vi "XIPIN_FIFO_Generator_13_0.vi"   [LabVIEW 2017]
doc: "The FIFO Generator is a parameterizable first-in/first-out memory queue generator. Use it to generate resource and performance optimized FIFOs with common or independent read/write clock domains, and optional fixed or programmable full and empty flags and handshaking signals. Choose from a selection of memory resource types for implementation. Optional Hamming code based error detection and correction as well as error injection capability for system test help to insure data integrity. FIFO width and depth are parameterizable, and for native interface FIFOs, asymmetric read and write port widths are also supported.\n------------------------------------\n<b>Need License</b> : No\n<b>Interface</b> : AXI4 AXI4-Stream"
uses:
  <vilib>/rvi/XilinxIP/XIPIN_XNode/niFpgaXIPIN.xnode
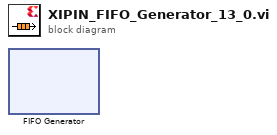
[diagram p0: block diagram]
diagram:
  n1 = xnode ("FIFO Generator")() -> ()
